vi "Register Tip Strip.vi"(8 "error in (no error)":errorcluster, 11 "Controls[]":refnum<vi>[](array[refnum])) -> (0 "error out":errorcluster)   [LabVIEW 2017]
doc: "Takes an array of FP controls and registers them to display a popup tip strip based on their tip strip text. best to turn off tip strips for the FP for which this is active, else you may get two tip strips popping up."
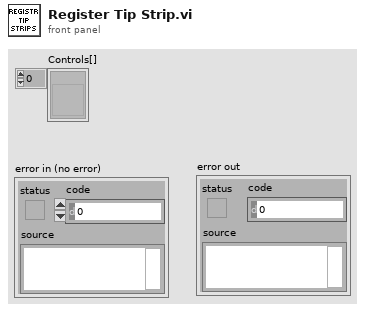
[diagram p1: front panel]
types:
  T1 = enum32{"Bad", "Idle", "Run top level", "Running"}
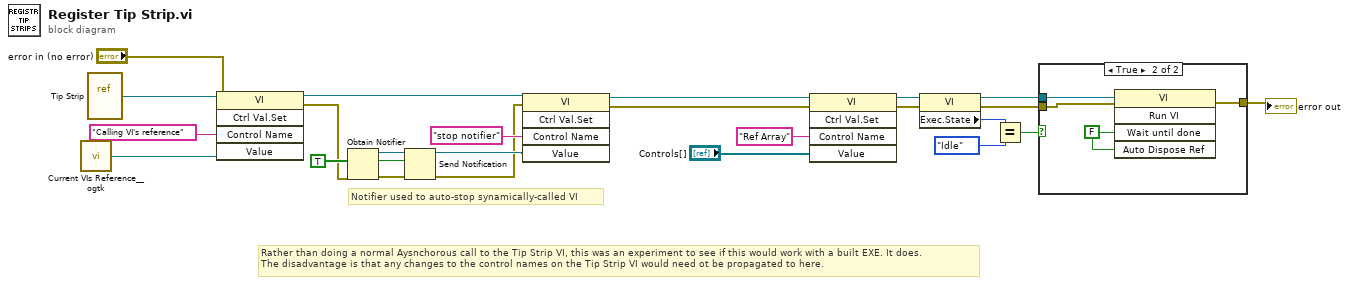
[diagram p0: block diagram]
diagram:
  w22 = TRUE
  # "Rather than doing a normal Aysnchorous call to the Tip Strip VI, this was an experiment to see if this would work with a built EXE. It does.\nThe disadvantage is that any changes to the control names on the Tip Strip VI would need ot be propagated to here."
  # "Notifier used to auto-stop synamically-called VI"
  n1 = call "Current VIs Reference__ogtk.vi"() -> ("Current VI's reference"=w2:refnum<vi>)  [unwired: 5 in]
  n2 = vi-ref "Tip Strip.vi"() -> (w11:refnum<vi>)
  n3 = invoke class="VI" method="Ctrl Val.Set"(reference=w11, error in="error in (no error)", "Control Name"="Calling VI's reference", "Value"=w2) -> (reference out=w10:refnum<vi>, error out=w7:errorcluster)  [unwired: 1 in, 3 out]
  n4 = Obtain Notifier(notification data type=w22, error in (no error)=w7) -> (notifier out=w20:refnum<notifier>, error out=w21:errorcluster)  [unwired: 2 in, 1 out]
  n5 = Send Notification(notification=w22, notifier=w20, error in (no error)=w21) -> (notifier out=w19:refnum<notifier>, error out=w6:errorcluster)
  n6 = invoke class="VI" method="Ctrl Val.Set"(reference=w10, error in=w6, "Control Name"="stop notifier", "Value"=w19) -> (reference out=w18:refnum<vi>, error out=w5:errorcluster)  [unwired: 1 in, 3 out]
  n7 = invoke class="VI" method="Ctrl Val.Set"(reference=w18, error in=w5, "Control Name"="Ref Array", "Value"="Controls[]") -> (reference out=w14:refnum<vi>, error out=w4:errorcluster)  [unwired: 1 in, 3 out]
  n8 = property class="VI"(reference=w14, error in=w4) -> (reference out=w13:refnum<vi>, error out=w3:errorcluster, "Exec.State"=w17:T1)
  n9 = Equal?(x=w17, y=T1."Idle" ("Execution:State")) -> (x = y?=w15:bool)
  n10 = case shown="True" w15 {
    tunnel: w13 -> [_ w28]
    tunnel: w3 -> [w25 w27]
    tunnel: [w25 w26] -> w1
    frame False {
    }
    frame True {
      w29 = FALSE
      n11 = invoke class="VI" method="Run VI"(reference=w28, error in=w27, "Wait until done"=w29, "Auto Dispose Ref"=w29) -> (error out=w26:errorcluster)  [unwired: 1 in, 4 out]
    }
  }
  "error out" <- w1
